vi "MB test.vi"() -> ()   [LabVIEW 2021]
uses:
  enums/DO.ctl
  enums/Param_MB test.lvlib
  enums/AO.ctl
  Inputs/Inputs.lvlib
  <vilib>/Platform/TimedLoop/XDataNode/XDataNode.xnode
  <vilib>/Platform/TimedLoop/XDataNode/nitl_modes.ctl
  <vilib>/Platform/TimedLoop/XDataNode/XDNodeRunTimeDep.lvlib
  <vilib>/Platform/TimedLoop/XDataNode/wakeup.ctl
  <vilib>/Platform/TimedLoop/XDataNode/timing_clust.ctl
  enums/AI.ctl
  enums/PAR.ctl
  enums/DI.ctl
  enums/DI_FAST.ctl
  enums/ALR.ctl
  enums/System.ctl
  enums/main_prog_state.ctl
  enums/KFM.ctl
  Userlib.lvlib
  OPC/OPC addons.lvlib
  Messages/Messages.lvlib
  enums/REG.ctl
  enums/supervisor_state.ctl
  Alarms/Alarms.lvlib
  enums/init_state.ctl
  enums/close_state.ctl
  MB/Modbus Master CR.lvclass
  PostgreSQL/Save messages PGserver/Save messages PGserver.lvclass
  Modbus_v121c/Data Model/Device Data Model.lvclass
panel:
  in  "DO2D":bool[][](array[boolean])
  in  "AOint":u16[][](array[numeric])
  out "Connect":bool[](array[boolean])
  in  "input Flags":T1={"write database started"=FALSE, "main prog started"=TRUE}
  out "output Flags":T2
  out "comm error":errorcluster
  out "initialise error":errorcluster
  in  "object_name":string="GM1"
  in  "EP_dist":bool
  in  "EP_on":bool
  in  "tick":i64=100 caption="Время цикла основной программы" min=5 max=500 step=1
  in  "stop":bool
  in  "On":bool=TRUE
  # "Включение записи !"
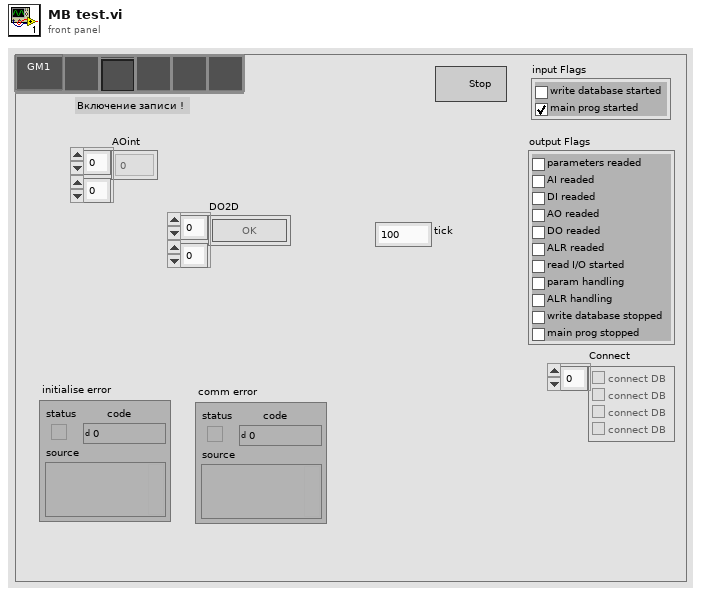
[diagram p1: front panel]
types:
  T1 = cluster{"write database started":bool, "main prog started":bool}
  T2 = cluster{"parameters readed ":bool, "AI readed":bool, "DI readed":bool, "AO readed":bool, "DO readed":bool, "ALR readed":bool, "read I/O started":bool, "param handling":bool, "ALR handling":bool, "write database stopped":bool, "main prog stopped":bool}
  T3 = typedef "Param_MB test.lvlib/init_state.ctl" = enum16{"Init Data", "Init TMPs", "Init system DB", "Init data DB", "Read Enums", "Init arrays", "Init KFM", "Init Param", "Init AI param", "Init DI param", "Init AO param", "Init DO param", "Init ALR param", "Init save progs", "Read OPC param", "Init Shared Variables", "Init regulators", "Init heaters", "Init Y defs", "Exit"}
  T4 = typedef "Param_MB test.lvlib/supervisor_state.ctl" = enum8{"initialize", "read parameters", "read AI param", "read DI param", "read AO param", "read DO param", "read ALR param", "write initialise param", "start read I/O modules", "wait for I/O start", "start param handling", "start ALR handling", "start write database", "start controls", "enable write outputs", "on", "off start", "disable write outputs", "stop controls", "stop write database", "wait for database stopped", "stop ALR handling", "stop param handling", "stop main prog", "stop read I/O modules", "wait for IO stop", "reset", "stop"}
  T5 = typedef "Param_MB test.lvlib/main_prog_state.ctl" = enum16{"Read_AI_Param", "Read_DI_Param", "Read_AO_Param", "Read_DO_Param", "Read_ALR_ON_OFF", "Read_ALR_Param", "Read_Param", "Read_REG_Param", "Timers", "AI", "DI", "SendAItoScada", "SendDItoScada", "Alarms", "SendAItoDB", "SendDItoDB", "SendALRtoDB", "Messages", "Controls", "Control HT1", "QN_control", "QN", "QN_state", "Control EB3", "Outputs", "Exit"}
  T6 = cluster{"KFM":string[], "PAR":string[], "AI":string[], "DI":string[], "DI_fast":string[], "AO":string[], "Regs":string[], "DO":string[], "ALR":string[], "System":string[]}
  T7 = cluster{"object_name":string, "Enums":cluster{"KFM":string[], "PAR":string[], "AI":string[], "DI":string[], "DI_fast":string[], "AO":string[], "Regs":string[], "DO":string[], "ALR":string[], "System":string[]}, "MBs":refnum<class "Modbus Master CR.lvclass">[]}
  T8 = cluster{"current time":timestamp, "Timer_1s":bool, "Timer_10s":bool, "Timer_1day":bool}
  T9 = typedef "Param_MB test.lvlib/REG.ctl" = enum16{"GM1QN1", "GM1QN2", "GM1QN3", "GM1QN4", "GM1QN5", "GM1QN6", "GM1QN7", "GM1QN8", "GM1QN9", "GM1QN10", "GM1QN11", "GM1QN12", "GM1QN13", "GM1QN14", "GM1QN15", "GM1QN16", "GM1QN17", "GM1QN18", "GM1QN19", "GM1QN20", "GM1QN21", "GM1QN22", "GM1QN23"}
  T10 = typedef "Param_MB test.lvlib/System.ctl" = enum16{"GM3HT1", "GM3HT2", "EB2TB1", "EB2TB2", "EB2TB3", "EB3TB1", "EB3TB2", "EB3TB3"}
  T11 = typedef "Param_MB test.lvlib/ALR.ctl" = enum16{"GM1BP1XQ01_H", "GM1BP1XQ01_HH", "GM1BP1XQ01_L", "GM1BP1XQ01_LL", "GM1BP1XQ01_SERR", "GM1BP2XQ01_H", "GM1BP2XQ01_HH", "GM1BP2XQ01_L", "GM1BP2XQ01_LL", "GM1BP2XQ01_SERR", "GM1BP3XQ01_H", "GM1BP3XQ01_HH", "GM1BP3XQ01_L", "GM1BP3XQ01_LL", "GM1BP3XQ01_SERR", "GM1BP4XQ01_H", "GM1BP4XQ01_HH", "GM1BP4XQ01_L", "GM1BP4XQ01_LL", "GM1BP4XQ01_SERR", "GM1BP5XQ01_H", "GM1BP5XQ01_HH", "GM1BP5XQ01_L", "GM1BP5XQ01_LL", "GM1BP5XQ01_SERR", "GM1BP6XQ01_H", "GM1BP6XQ01_HH", "GM1BP6XQ01_L", "GM1BP6XQ01_LL", "GM1BP6XQ01_SERR", "GM1BT1XQ01_H", "GM1BT1XQ01_HH", "GM1BT1XQ01_L", "GM1BT1XQ01_SERR", "GM1BT2XQ01_H", "GM1BT2XQ01_HH", "GM1BT2XQ01_L", "GM1BT2XQ01_SERR", "GM1BT3XQ01_H", "GM1BT3XQ01_HH", "GM1BT3XQ01_L", "GM1BT3XQ01_SERR", "GM1BT4XQ01_H", "GM1BT4XQ01_HH", "GM1BT4XQ01_L", "GM1BT4XQ01_SERR", "GM1BT5XQ01_H", "GM1BT5XQ01_HH", "GM1BT5XQ01_L", "GM1BT5XQ01_SERR", "GM1BT6XQ01_H", "GM1BT6XQ01_HH", "GM1BT6XQ01_L", "GM1BT6XQ01_SERR", "GM1BT7XQ01_H", "GM1BT7XQ01_HH", "GM1BT7XQ01_L", "GM1BT7XQ01_SERR", "GM1BT8XQ01_H", "GM1BT8XQ01_HH", "GM1BT8XQ01_L", "GM1BT8XQ01_SERR", "GM1BT9XQ01_H", "GM1BT9XQ01_HH", "GM1BT9XQ01_L", "GM1BT9XQ01_SERR", "GM1BT10XQ01_H", "GM1BT10XQ01_HH", "GM1BT10XQ01_L", "GM1BT10XQ01_SERR", "GM1BT19XQ01_H", "GM1BT19XQ01_HH", "GM1BT19XQ01_L", "GM1BT19XQ01_SERR", "GM1BT20XQ01_H", "GM1BT20XQ01_HH", "GM1BT20XQ01_L", "GM1BT20XQ01_SERR", "GM1BT21XQ01_H", "GM1BT21XQ01_HH", "GM1BT21XQ01_L", "GM1BT21XQ01_SERR", "GM1BT22XQ01_H", "GM1BT22XQ01_HH", "GM1BT22XQ01_L", "GM1BT22XQ01_SERR", "GM1QN1XQ01_SERR", "GM1QN1XQ02_HH", "GM1QN2XQ01_SERR", "GM1QN2XQ02_HH", "GM1QN3XQ01_SERR", "GM1QN3XQ02_HH", "GM1QN4XQ01_SERR", "GM1QN4XQ02_HH", "GM1QN5XQ01_SERR", "GM1QN5XQ02_HH", "GM1QN6XQ01_SERR", "GM1QN6XQ02_HH", "GM1QN7XQ01_SERR", "GM1QN7XQ02_HH", "GM1QN8XQ01_SERR", "GM1QN8XQ02_HH", "GM1QN9XQ01_SERR", "GM1QN9XQ02_HH", "GM1QN10XQ01_SERR", "GM1QN10XQ02_HH", "GM1QN11XQ01_SERR", "GM1QN11XQ02_HH", "GM1QN12XQ01_SERR", "GM1QN12XQ02_HH", "GM1QN13XQ01_SERR", "GM1QN13XQ02_HH", "GM1QN14XQ01_SERR", "GM1QN14XQ02_HH", "GM1QN15XQ01_SERR", "GM1QN15XQ02_HH", "GM1QN16XQ01_SERR", "GM1QN16XQ02_HH", "GM1QN17XQ01_SERR", "GM1QN17XQ02_HH", "GM1QN18XQ01_SERR", "GM1QN18XQ02_HH", "GM1QN19XQ01_SERR", "GM1QN19XQ02_HH", "GM1QN20XQ01_SERR", "GM1QN20XQ02_HH", "GM1QN21XQ01_SERR", "GM1QN21XQ02_HH", "GM1QN22XQ01_SERR", "GM1QN22XQ02_HH", "GM1QN23XQ01_SERR", "GM1QN23XQ02_HH", "HX1BT11XQ01_H", "HX1BT11XQ01_HH", "HX1BT11XQ01_L", "HX1BT11XQ01_SERR", "HX1BT12XQ01_H", "HX1BT12XQ01_HH", "HX1BT12XQ01_L", "HX1BT12XQ01_SERR", "HX1BT21XQ01_H", "HX1BT21XQ01_HH", "HX1BT21XQ01_L", "HX1BT21XQ01_SERR", "HX1BT22XQ01_H", "HX1BT22XQ01_HH", "HX1BT22XQ01_L", "HX1BT22XQ01_SERR", "HX1BT31XQ01_H", "HX1BT31XQ01_HH", "HX1BT31XQ01_L", "HX1BT31XQ01_SERR", "HX1BT32XQ01_H", "HX1BT32XQ01_HH", "HX1BT32XQ01_L", "HX1BT32XQ01_SERR", "HX1BT41XQ01_H", "HX1BT41XQ01_HH", "HX1BT41XQ01_L", "HX1BT41XQ01_SERR", "HX1BT42XQ01_H", "HX1BT42XQ01_HH", "HX1BT42XQ01_L", "HX1BT42XQ01_SERR", "GM1JBA1JA1_CONN", "GM1JBA1JA2_CONN", "GM1JBA2JA1_CONN", "GM1JBA2JA2_CONN", "GM1JBA3JA1_CONN", "HX1KF1A16_CONN", "HX1KF1A17_CONN", "GM1KF1A18_CONN"}
  T12 = typedef "Param_MB test.lvlib/DO.ctl" = enum16{"GM1FZ1_YB47"}
  T13 = typedef "Param_MB test.lvlib/AO.ctl" = enum16{"GM1QN1_YQ01", "GM1QN2_YQ01", "GM1QN3_YQ01", "GM1QN4_YQ01", "GM1QN5_YQ01", "GM1QN6_YQ01", "GM1QN7_YQ01", "GM1QN8_YQ01", "GM1QN9_YQ01", "GM1QN10_YQ01", "GM1QN11_YQ01", "GM1QN12_YQ01", "GM1QN13_YQ01", "GM1QN14_YQ01", "GM1QN15_YQ01", "GM1QN16_YQ01", "GM1QN17_YQ01", "GM1QN18_YQ01", "GM1QN19_YQ01", "GM1QN20_YQ01", "GM1QN21_YQ01", "GM1QN22_YQ01", "GM1QN23_YQ01"}
  T14 = typedef "Param_MB test.lvlib/DI_FAST.ctl" = enum16{"W1.KF_XB01", "W1.KF_XB02", "W1.KF_XB03", "W1.KF_XB04", "W1.KF_XB05", "W1.KF_XB06", "W1.KF_XB07", "W1.KF_XB08", "W1.KF_XB09", "W1.KF_XB10", "W1.KF_XB11", "W1.KF_XB12", "W1.KF_XB13", "W1.KF_XB14", "W1.KF_XB15", "W1.KF_XB16"}
  T15 = typedef "Param_MB test.lvlib/DI.ctl" = enum16{"GM1FZ1_XB19"}
  T16 = typedef "Param_MB test.lvlib/AI.ctl" = enum16{"GM1BP1_XQ01", "GM1BP2_XQ01", "GM1BP3_XQ01", "GM1BP4_XQ01", "GM1BP5_XQ01", "GM1BP6_XQ01", "GM1BT1_XQ01", "GM1BT2_XQ01", "GM1BT3_XQ01", "GM1BT4_XQ01", "GM1BT5_XQ01", "GM1BT6_XQ01", "GM1BT7_XQ01", "GM1BT8_XQ01", "GM1BT9_XQ01", "GM1BT10_XQ01", "GM1BT19_XQ01", "GM1BT20_XQ01", "HX1BT11_XQ01", "HX1BT12_XQ01", "HX1BT21_XQ01", "HX1BT22_XQ01", "HX1BT31_XQ01", "HX1BT32_XQ01", "HX1BT41_XQ01", "HX1BT42_XQ01", "GM1QN1_XQ01", "GM1QN2_XQ01", "GM1QN3_XQ01", "GM1QN4_XQ01", "GM1QN5_XQ01", "GM1QN6_XQ01", "GM1QN7_XQ01", "GM1QN8_XQ01", "GM1QN9_XQ01", "GM1QN10_XQ01", "GM1QN11_XQ01", "GM1QN12_XQ01", "GM1QN13_XQ01", "GM1QN14_XQ01", "GM1QN15_XQ01", "GM1QN16_XQ01", "GM1QN17_XQ01", "GM1QN18_XQ01", "GM1QN19_XQ01", "GM1QN20_XQ01", "GM1QN21_XQ01", "GM1QN22_XQ01", "GM1QN23_XQ01", "GM1QN1_XQ02", "GM1QN2_XQ02", "GM1QN3_XQ02", "GM1QN4_XQ02", "GM1QN5_XQ02", "GM1QN6_XQ02", "GM1QN7_XQ02", "GM1QN8_XQ02", "GM1QN9_XQ02", "GM1QN10_XQ02", "GM1QN11_XQ02", "GM1QN12_XQ02", "GM1QN13_XQ02", "GM1QN14_XQ02", "GM1QN15_XQ02", "GM1QN16_XQ02", "GM1QN17_XQ02", "GM1QN18_XQ02", "GM1QN19_XQ02", "GM1QN20_XQ02", "GM1QN21_XQ02", "GM1QN22_XQ02", "GM1QN23_XQ02", "GM1BT21_XQ01", "GM1BT22_XQ01"}
  T17 = typedef "Param_MB test.lvlib/PAR.ctl" = enum16{"GM1QN1_alr_value", "GM1QN1_auto_value", "GM1QN1_output_set_time", "GM1QN1_group", "GM1QN1_process_gas", "GM1QN2_alr_value", "GM1QN2_auto_value", "GM1QN2_output_set_time", "GM1QN2_group", "GM1QN2_process_gas", "GM1QN3_alr_value", "GM1QN3_auto_value", "GM1QN3_output_set_time", "GM1QN3_group", "GM1QN3_process_gas", "GM1QN4_alr_value", "GM1QN4_auto_value", "GM1QN4_output_set_time", "GM1QN4_group", "GM1QN4_process_gas", "GM1QN5_alr_value", "GM1QN5_auto_value", "GM1QN5_output_set_time", "GM1QN5_group", "GM1QN5_process_gas", "GM1QN6_alr_value", "GM1QN6_auto_value", "GM1QN6_output_set_time", "GM1QN6_group", "GM1QN6_process_gas", "GM1QN7_alr_value", "GM1QN7_auto_value", "GM1QN7_output_set_time", "GM1QN7_group", "GM1QN7_process_gas", "GM1QN8_alr_value", "GM1QN8_auto_value", "GM1QN8_output_set_time", "GM1QN8_group", "GM1QN8_process_gas", "GM1QN9_alr_value", "GM1QN9_auto_value", "GM1QN9_output_set_time", "GM1QN9_group", "GM1QN9_process_gas", "GM1QN10_alr_value", "GM1QN10_auto_value", "GM1QN10_output_set_time", "GM1QN10_group", "GM1QN10_process_gas", "GM1QN11_alr_value", "GM1QN11_auto_value", "GM1QN11_output_set_time", "GM1QN11_group", "GM1QN11_process_gas", "GM1QN12_alr_value", "GM1QN12_auto_value", "GM1QN12_output_set_time", "GM1QN12_group", "GM1QN12_process_gas", "GM1QN13_alr_value", "GM1QN13_auto_value", "GM1QN13_output_set_time", "GM1QN13_group", "GM1QN13_process_gas", "GM1QN14_alr_value", "GM1QN14_auto_value", "GM1QN14_output_set_time", "GM1QN14_group", "GM1QN14_process_gas", "GM1QN15_alr_value", "GM1QN15_auto_value", "GM1QN15_output_set_time", "GM1QN15_group", "GM1QN15_process_gas", "GM1QN16_alr_value", "GM1QN16_auto_value", "GM1QN16_output_set_time", "GM1QN16_group", "GM1QN16_process_gas", "GM1QN17_alr_value", "GM1QN17_auto_value", "GM1QN17_output_set_time", "GM1QN17_group", "GM1QN17_process_gas", "GM1QN18_alr_value", "GM1QN18_auto_value", "GM1QN18_output_set_time", "GM1QN18_group", "GM1QN18_process_gas", "GM1QN19_alr_value", "GM1QN19_auto_value", "GM1QN19_output_set_time", "GM1QN19_group", "GM1QN19_process_gas", "GM1QN20_alr_value", "GM1QN20_auto_value", "GM1QN20_output_set_time", "GM1QN20_group", "GM1QN20_process_gas", "GM1QN21_alr_value", "GM1QN21_auto_value", "GM1QN21_output_set_time", "GM1QN21_group", "GM1QN21_process_gas", "GM1QN22_alr_value", "GM1QN22_auto_value", "GM1QN22_output_set_time", "GM1QN22_group", "GM1QN22_process_gas", "GM1QN23_alr_value", "GM1QN23_auto_value", "GM1QN23_output_set_time", "GM1QN23_group", "GM1QN23_process_gas"}
  T18 = typedef "Param_MB test.lvlib/KFM.ctl" = enum16{"GM1KF1_A1", "GM1JBA1_JA1", "GM1JBA1_JA2", "GM1JBA2_JA1", "GM1JBA2_JA2", "GM1JBA3_JA1", "HX1KF1_A16", "HX1KF1_A17", "GM1KF1_A18"}
  T19 = typedef "XDNodeRunTimeDep.lvlib/timing_clust.ctl" = cluster{"Expected End [f-1]":u64, "Actual End [f-1]":u64, "Finished Late? [f-1]":bool, "Expected End [i-1]":u64, "Actual End [i-1]":u64, "Finished Late? [i-1]":bool, "Expected Start [i]":u64, "Actual Start [i]":u64, "Expected Start [f]":u64, "Actual Start [f]":u64, "Source Name":string, "Structure Name":string, "Period":i64, "Deadline":i64, "Offset":i64, "Start":i64, "Priority":i32, "Timeout":i32, "Mode":T20, "Wakeup Reason":T21, "Error":errorcluster, "Source Type":string, "Secondary Source Type":string, "Global End Time":u64, "Global Start Time":u64, "Frame Duration":u64, "Iteration Duration":u64, "Assigned CPU":i32, "I/O Scan Engine Mode":u32}
  T20 = typedef "XDNodeRunTimeDep.lvlib/nitl_modes.ctl" = enum32{"No Change", "Process missed periods, maintain original phase", "Discard missed periods, maintain original phase", "Process missed periods, ignore original phase", "Discard missed periods, ignore original phase"}
  T21 = typedef "XDNodeRunTimeDep.lvlib/wakeup.ctl" = enum32{"Normal", "Aborted", "Asynchronous wakeup", "Timing source error", "Timed loop error", "Timeout"}
  T22 = typedef "MB_v2.lvlib/Modbus Master CR.lvclass/N channel.ctl" = cluster{"N DI channel":u16, "N DO channel":u16, "N AI channel":u16, "N AO channel":u16}
  T23 = typedef "Param_MB test.lvlib/close_state.ctl" = enum16{"QN_state notifier", "QN_control_queue", "ALR notifires", "ALR", "DO notifires", "DO", "AO notifires", "AO", "DI notifres", "DI", "AI notifires", "AI", "OPC", "Param", "SaveMessageProg", "KFM DadaRef", "KFM Registers", "KFM StatusRef", "Exit"}
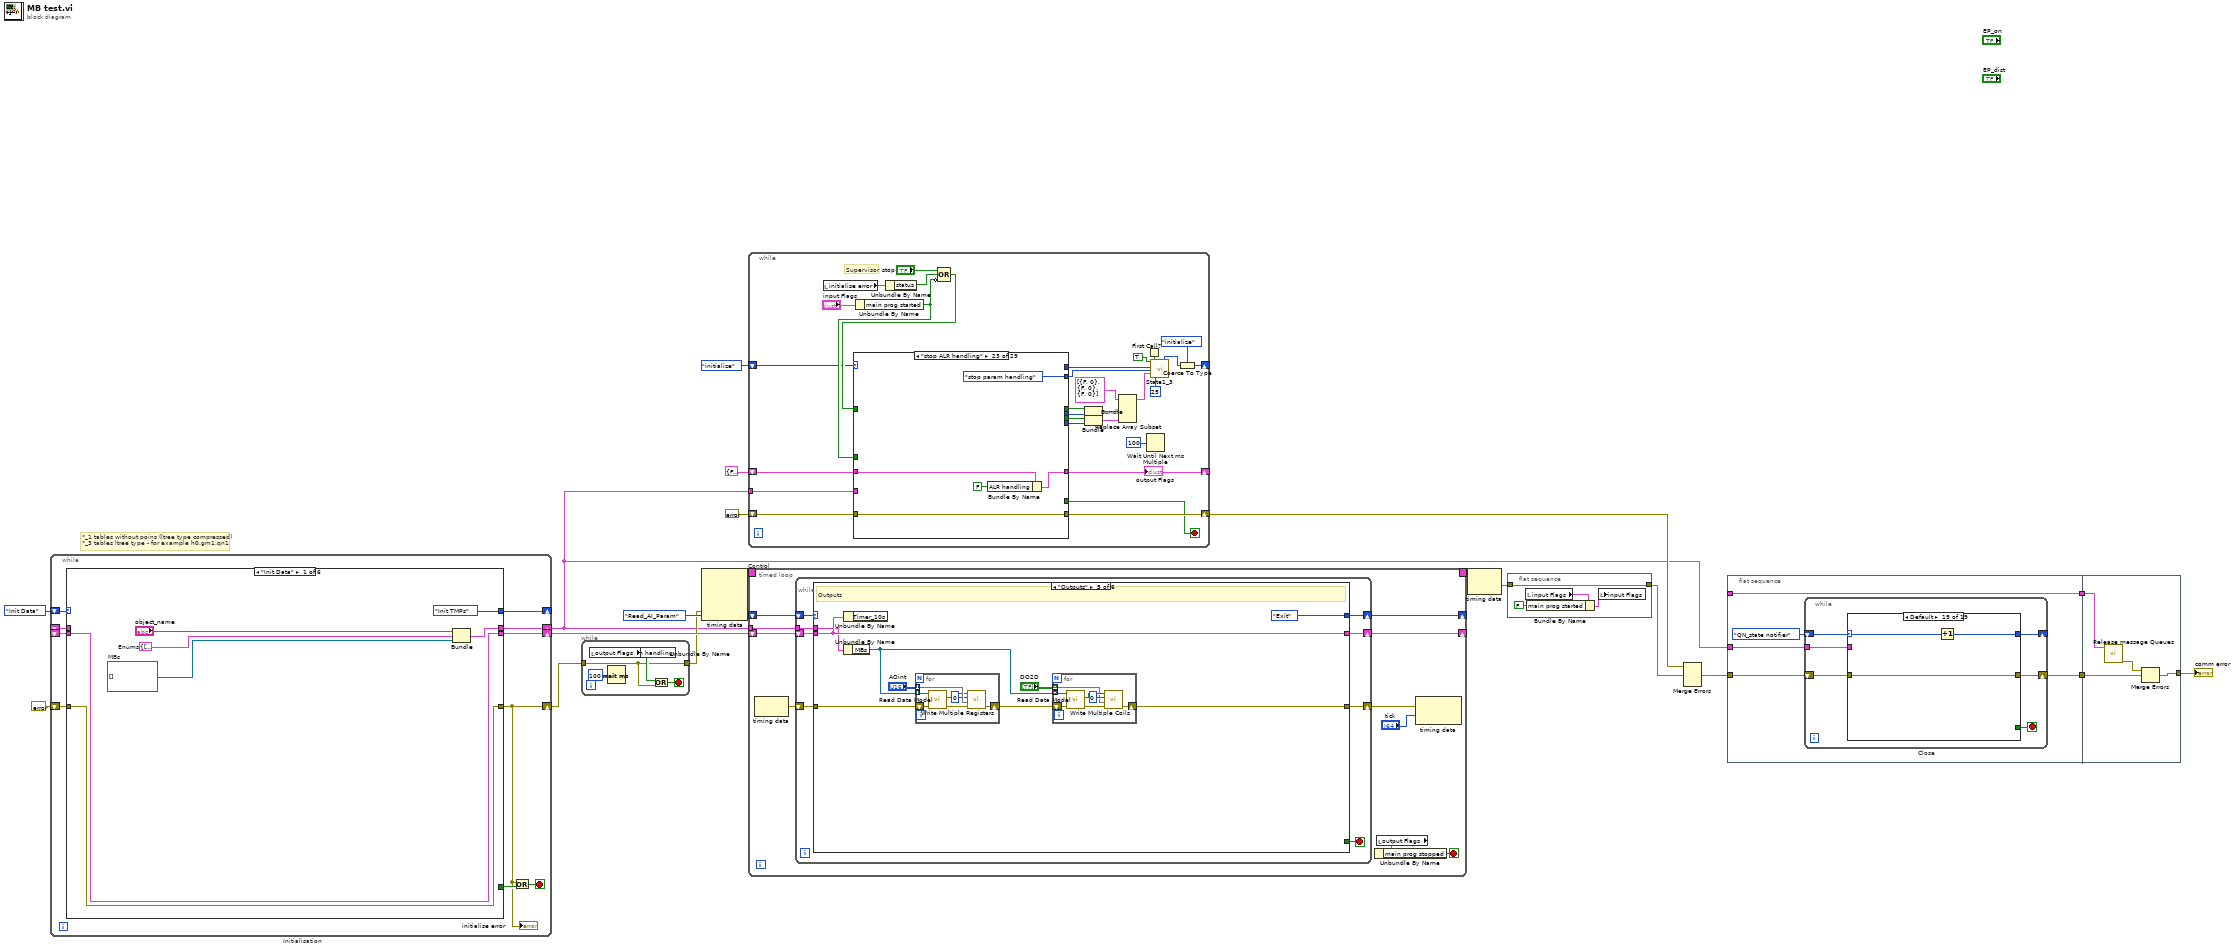
[diagram p0: block diagram]
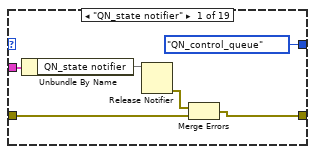
[diagram p2: hidden frame]
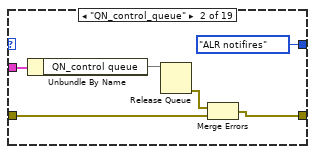
[diagram p3: hidden frame]
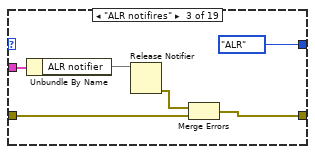
[diagram p4: hidden frame]
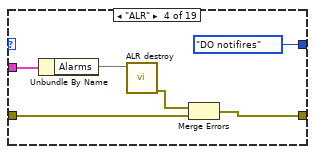
[diagram p5: hidden frame]
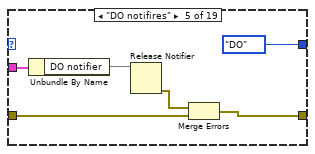
[diagram p6: hidden frame]
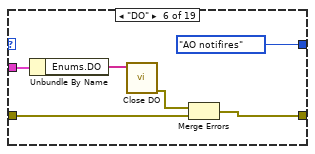
[diagram p7: hidden frame]
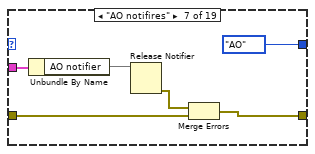
[diagram p8: hidden frame]
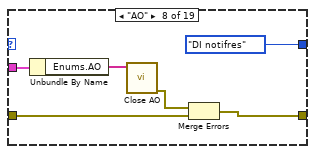
[diagram p9: hidden frame]
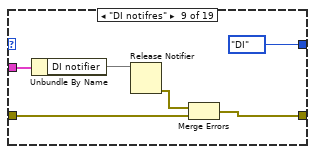
[diagram p10: hidden frame]
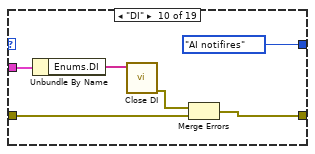
[diagram p11: hidden frame]
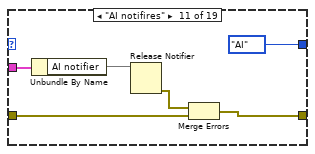
[diagram p12: hidden frame]
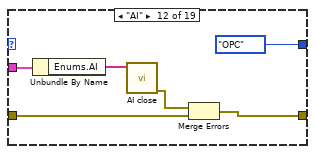
[diagram p13: hidden frame]
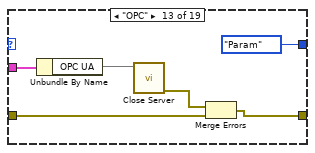
[diagram p14: hidden frame]
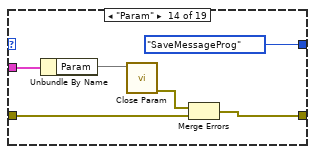
[diagram p15: hidden frame]
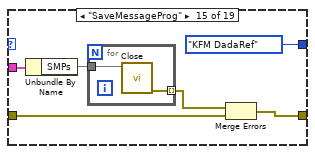
[diagram p16: hidden frame]
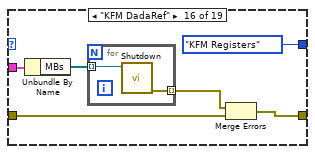
[diagram p17: hidden frame]
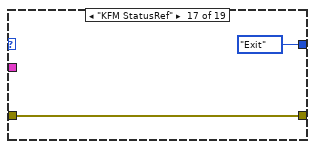
[diagram p18: hidden frame]
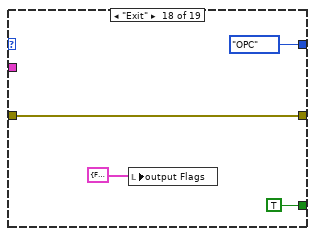
[diagram p19: hidden frame]
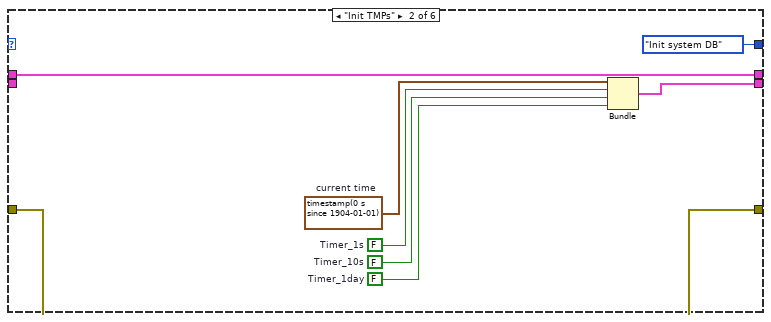
[diagram p20: hidden frame]
diagram:
  # "*_1 tables without poins (ltree type compressed)\n*_3 tables ltree type - for example h0.gm1.qn1"
  n1 = while "Initialisation" {
    shift-right: [w20] -> w9
    shift-left: errorcluster {"status"=FALSE, "code"=0, "source"=""} ("error out") -> [w26]
    shift-right: [w29] -> w2
    shift-left: _ -> [w27]
    shift-right: [w25] -> _
    shift-left: init_state."Init Data" -> [w28]
    shift-right: [w22] -> w10
    shift-left: _ -> [w21]
    stop <- w23 stop-if-true
    # "Initialisation"
    n2 = case shown="\"Init Data\"" w28 {
      tunnel: [w34 w43 w61 w83 w101 w104] -> w20
      selector: w28 -> [_ _ _ _ _ w107]
      tunnel: [w35 w42 w78 w88 w102 w105] -> w29
      tunnel: w27 -> [_ w42 w79 w87 w102 w105]
      tunnel: w26 -> [w34 w43 w45 w84 w101 w104]
      tunnel: [init_state."Init TMPs" init_state."Init system DB" init_state."Init arrays" init_state."Init Param" init_state."Init Data" w106] -> w25
      tunnel: [_ _ _ _ TRUE _] -> w24
      tunnel: [w32 w41 w81 w94 w99 w108] -> w22
      tunnel: w21 -> [w32 _ w81 w94 w99 w108]
      frame "Init Data" {
        w30 = refnum<class "Modbus Master CR.lvclass">[] []  # MBs
        w33 = T6 {"KFM"=[], "PAR"=[], "AI"=[], "DI"=[], "DI_fast"=[], "AO"=[], "Regs"=[], "DO"=[], "ALR"=[], "System"=[]}  # Enums
        n3 = Bundle("object_name"="object_name", "Enums"=w33, "MBs"=w30) -> (w35:T7)  [unwired: 1 in]
      }
      frame "Init TMPs" {
        w37 = FALSE  # Timer_10s
        w38 = FALSE  # Timer_1day
        w39 = FALSE  # Timer_1s
        w40 = timestamp(0 s since 1904-01-01)  # current time
        n4 = Bundle("current time"=w40, "Timer_1s"=w39, "Timer_10s"=w37, "Timer_1day"=w38) -> (w41:T8)  [unwired: 1 in]
      }
      frame "Read Enums" {
        w47 = REG."GM1QN1"  # REG
        w50 = T6 {"KFM"=[], "PAR"=[], "AI"=[], "DI"=[], "DI_fast"=[], "AO"=[], "Regs"=[], "DO"=[], "ALR"=[], "System"=[]}  # Enums
        w52 = System."GM3HT1"  # System_enum
        w53 = ALR."GM1JBA1JA1_CONN"  # ALR_enum
        w54 = DO."GM1FZ1_YB47"  # DO_enum
        w55 = AO."GM1QN1_YQ01"  # AO_enum
        w56 = DI_FAST."W1.KF_XB01"  # DI_enum fast
        w57 = DI."GM1FZ1_XB19"  # DI_enum
        w58 = AI."GM1QN1_XQ01"  # AI_enum
        w59 = PAR."GM1QN1_output_set_time"  # PAR_enum
        w60 = KFM."GM1JBA1_JA1"  # KFM_enum
        # "компьютер на 0 месте"
        n5 = call <userlib>:"Get Strings from Enum__ogtk.vi"("error in (no error)"=w45, "Enum"=w60) -> ("error out"=w70:errorcluster, "Enum Strings"=w77:string[])  [unwired: 6 in, 2 out]
        n6 = call <userlib>:"Get Strings from Enum__ogtk.vi"("error in (no error)"=w45, "Enum"=w59) -> ("error out"=w69:errorcluster, "Enum Strings"=w76:string[])  [unwired: 6 in, 2 out]
        n7 = call <userlib>:"Get Strings from Enum__ogtk.vi"("error in (no error)"=w45, "Enum"=w58) -> ("error out"=w68:errorcluster, "Enum Strings"=w75:string[])  [unwired: 6 in, 2 out]
        n8 = call <userlib>:"Get Strings from Enum__ogtk.vi"("error in (no error)"=w45, "Enum"=w57) -> ("error out"=w67:errorcluster, "Enum Strings"=w74:string[])  [unwired: 6 in, 2 out]
        n9 = call <userlib>:"Get Strings from Enum__ogtk.vi"("error in (no error)"=w45, "Enum"=w56) -> ("error out"=w66:errorcluster, "Enum Strings"=w73:string[])  [unwired: 6 in, 2 out]
        n10 = call <userlib>:"Get Strings from Enum__ogtk.vi"("error in (no error)"=w45, "Enum"=w55) -> ("error out"=w65:errorcluster, "Enum Strings"=w72:string[])  [unwired: 6 in, 2 out]
        n11 = call <userlib>:"Get Strings from Enum__ogtk.vi"("error in (no error)"=w45, "Enum"=w47) -> ("Enum Strings"=w46:string[])  [unwired: 6 in, 3 out]
        n12 = call <userlib>:"Get Strings from Enum__ogtk.vi"("error in (no error)"=w45, "Enum"=w54) -> ("error out"=w64:errorcluster, "Enum Strings"=w48:string[])  [unwired: 6 in, 2 out]
        n13 = call <userlib>:"Get Strings from Enum__ogtk.vi"("error in (no error)"=w45, "Enum"=w53) -> ("error out"=w63:errorcluster, "Enum Strings"=w71:string[])  [unwired: 6 in, 2 out]
        n14 = call <userlib>:"Get Strings from Enum__ogtk.vi"("error in (no error)"=w45, "Enum"=w52) -> ("error out"=w62:errorcluster)  [unwired: 6 in, 3 out]
        n15 = Bundle By Name(cluster=w50, "KFM"=w77, "PAR"=w76, "AI"=w75, "DI"=w74, "DI_fast"=w73, "AO"=w72, "Regs"=w46, "DO"=w48, "ALR"=w71, "System"=string[] []) -> (w49:T6)
        n16 = Merge Errors(w70, w69, w68, w67, w66, w65, w64, w63, w62) -> (w61:errorcluster)
        n17 = Bundle By Name(cluster=w79, "Enums"=w49) -> (w78:T7)
      }
      frame "Init KFM" {
        n18 = Unbundle By Name(w87) -> ("Enums.KFM"=w91:string[])
        n19 = call "init classes.vi"("error in (no error)"=w84, "MVINames"=string[] []) -> ("error out"=w93:errorcluster, "MBs"=w85:refnum<class "Modbus Master CR.lvclass">[])  [unwired: 8 in]
        n20 = call "MB Param redefine.vi"("error in (no error)"=w93, "KFMTable"="kfm_1", "KFM param"=w91, "MBs"=w85) -> ("error"=w92:errorcluster, "MBs out"=w89:refnum<class "Modbus Master CR.lvclass">[])  [unwired: 6 in]
        n21 = call "Start read modules.vi"("error in"=w92, "classes"=w89) -> ("error out"=w83:errorcluster, "classes initialised"=w86:refnum<class "Modbus Master CR.lvclass">[])  [unwired: 8 in]
        n22 = Bundle By Name(cluster=w87, "MBs"=w86) -> (w88:T7)
      }
      frame "Exit" {
        n23 = local read "input Flags"() -> (w98:T1)
        n24 = Bundle By Name(cluster=w98, "main prog started"=TRUE) -> (w97:T1)
        n25 = local write "input Flags"(w97) -> ()
      }
      frame Default {
        n26 = Increment(x=w107) -> (x+1=w106:T3)
      }
    }
    "initialise error" <- w20
    n27 = Or(x=w20, y=w24) -> (x .or. y?=w23:bool)
  }
  n28 = while {
    tunnel: w9 -> [w110]
    tunnel: [w110] -> w8
    stop <- w109 stop-if-true
    n29 = local read "output Flags"() -> (w113:T2)
    n30 = Wait (ms)(milliseconds to wait=u32 100) -> ()  [unwired: 1 out]
    n31 = Unbundle By Name(w113) -> ("param handling"=w112:bool)
    n32 = Or(x=w112, y=w110) -> (x .or. y?=w109:bool)
  }
  n33 = node-c288(w8) -> (w19:T19)  [unwired: 3 in]
  n34 = while {
    tunnel: w2 -> [w125]
    shift-right: [w121] -> _
    shift-left: T2 {"parameters readed "=FALSE, "AI readed"=FALSE, "DI readed"=FALSE, "AO readed"=FALSE, "DO readed"=FALSE, "ALR readed"=FALSE, "read I/O started"=FALSE, "param handling"=FALSE, "ALR handling"=FALSE, "write database stopped"=FALSE, "main prog stopped"=FALSE} ("output Flags") -> [w126]
    shift-right: [w123] -> w7
    shift-left: errorcluster {"status"=FALSE, "code"=0, "source"=""} ("error out") -> [w124]
    shift-right: [w132] -> _
    shift-left: supervisor_state."initialize" ("Z2(SetState)") -> [w114]
    stop <- w122 stop-if-true
    # "Supervisor"
    n35 = local read "initialise error"() -> (w130:errorcluster)
    n36 = Unbundle By Name("input Flags") -> ("main prog started"=w127:bool)
    n37 = Unbundle By Name(w130) -> ("status"=w142:bool)
    n38 = Compound Arithmetic op=OR("stop", w142, invert w127) -> (w128:bool)
    n39 = case shown="\"stop ALR handling\"" w114 {
      selector: w114 -> [w145 _ _ _ _ _ _ _ _ _ _ _ _ _ _ _ _ _ _ _ _ _ _ _ _ _ _ _ _]
      tunnel: [_ _ w170 w184 w198 w212 w226 w240 _ w256 w275 w283 w290 w299 w305 w314 w328 _ _ _ _ _ _ _ _ _ _ _ _] -> w117
      tunnel: [_ _ supervisor_state."off start" ("Z2(SetState)") supervisor_state."off start" ("Z2(SetState)") supervisor_state."off start" ("Z2(SetState)") supervisor_state."off start" ("Z2(SetState)") supervisor_state."off start" ("Z2(SetState)") supervisor_state."off start" ("Z2(SetState)") _ supervisor_state."off start" ("Z2(SetState)") supervisor_state."off start" ("Z2(SetState)") supervisor_state."off start" ("Z2(SetState)") supervisor_state."off start" ("Z2(SetState)") supervisor_state."off start" ("Z2(SetState)") supervisor_state."off start" ("Z2(SetState)") supervisor_state."off start" ("Z2(SetState)") supervisor_state."off start" ("Z2(SetState)") _ _ _ _ _ _ _ _ _ _ _ _] -> w118
      tunnel: [u32 0 ("T") u32 0 ("T") u32 60000 ("T") u32 60000 ("T") u32 60000 ("T") u32 60000 ("T") u32 60000 ("T") u32 60000 ("T") _ _ u32 10000 ("T") u32 5000 ("T") _ _ u32 100 ("T") _ _ _ _ _ _ u32 60000 ("T") _ _ _ _ u32 10000 ("T") u32 2000 ("T") _] -> w115
      tunnel: [w144 supervisor_state."read parameters" ("Z2(SetState)") supervisor_state."read AI param" ("Z2(SetState)") supervisor_state."read DI param" ("Z2(SetState)") supervisor_state."read AO param" ("Z2(SetState)") supervisor_state."read DO param" ("Z2(SetState)") supervisor_state."read ALR param" ("Z2(SetState)") supervisor_state."start read I/O modules" ("Z2(SetState)") supervisor_state."start read I/O modules" ("Z2(SetState)") supervisor_state."wait for I/O start" ("Z2(SetState)") supervisor_state."start param handling" ("Z2(SetState)") supervisor_state."start ALR handling" ("Z2(SetState)") supervisor_state."start write database" ("Z2(SetState)") supervisor_state."start controls" ("Z2(SetState)") supervisor_state."enable write outputs" ("Z2(SetState)") supervisor_state."on" ("Z2(SetState)") supervisor_state."on" ("Z2(SetState)") supervisor_state."disable write outputs" ("Z2(SetState)") supervisor_state."stop controls" ("Z2(SetState)") supervisor_state."stop write database" ("Z2(SetState)") w355 w365 supervisor_state."stop param handling" ("Z2(SetState)") supervisor_state."stop main prog" ("Z2(SetState)") supervisor_state."stop main prog" ("Z2(SetState)") supervisor_state."wait for IO stop" ("Z2(SetState)") w398 supervisor_state."stop" ("Z2(SetState)") supervisor_state."stop" ("Z2(SetState)")] -> w116
      tunnel: [_ _ w160 w178 w192 w206 w220 w230 _ _ w267 _ _ _ _ _ _ _ _ _ _ w360 _ _ w381 _ w399 _ _] -> w119
      tunnel: [_ _ supervisor_state."read AI param" ("Z2(SetState)") supervisor_state."read DI param" ("Z2(SetState)") supervisor_state."read AO param" ("Z2(SetState)") supervisor_state."read DO param" ("Z2(SetState)") supervisor_state."read ALR param" ("Z2(SetState)") supervisor_state."start read I/O modules" ("Z2(SetState)") _ _ supervisor_state."start param handling" ("Z2(SetState)") _ _ _ _ _ _ _ _ _ w355 w365 _ _ supervisor_state."stop read I/O modules" ("Z2(SetState)") _ w398 _ _] -> w120
      tunnel: w128 -> [_ _ w170 w184 w198 w212 w226 w240 _ w256 w275 w283 w290 w299 w305 w314 w328 _ _ _ _ _ _ _ _ _ _ _ _]
      tunnel: [w148 w157 w161 w179 w193 w207 w221 w231 w246 w254 w264 w279 w287 w298 w303 w313 w327 w337 w344 w347 w353 w361 w368 w373 w378 w391 w401 w404 w408] -> w121
      tunnel: w126 -> [w148 w157 w163 w181 w195 w209 w223 w235 w246 w254 w263 w278 w286 w298 w303 w313 w327 w337 w344 w347 w353 w362 w367 w372 w377 w391 w401 w404 w408]
      tunnel: w124 -> [w147 w154 w165 w177 w191 w205 w219 w234 w245 w249 w262 w281 w289 w295 w302 w310 w324 w336 w340 w346 w352 w356 w370 w375 w383 w386 w394 w403 w407]
      tunnel: [w147 w150 w164 w175 w190 w204 w217 w232 w245 w247 w259 w281 w289 w294 w302 w308 w320 w336 w341 w346 w350 w359 w370 w375 w383 w385 w393 w403 w407] -> w123
      tunnel: w125 -> [_ w156 w162 w180 w194 w208 w222 w233 _ w255 w272 _ _ w297 _ w312 w325 _ w343 _ w354 w364 _ _ _ w389 w396 _ _]
      tunnel: w127 -> [_ _ _ _ _ _ _ _ _ _ _ _ _ _ _ _ _ _ _ _ _ _ _ _ w380 _ _ _ _]
      tunnel: [_ _ _ _ _ _ _ _ _ _ _ _ _ _ _ _ _ _ _ _ _ _ _ _ _ _ _ _ TRUE] -> w122
      frame Default {
        n40 = Increment(x=w145) -> (x+1=w144:T4)
      }
      frame "initialize" {
        n41 = Unbundle By Name(w156) -> ("MBs"=w155:refnum<class "Modbus Master CR.lvclass">[])
        n42 = call "Send Run.vi"("error in"=w154, "Run"=FALSE, "MBs"=w155) -> ("error out"=w151:errorcluster, "MBs out"=w152:refnum<class "Modbus Master CR.lvclass">[])  [unwired: 7 in]
        n43 = call "Send Write.vi"("error in"=w151, "Write"=FALSE, "MBs"=w152) -> ("error out"=w150:errorcluster)  [unwired: 7 in, 1 out]
      }
      frame "read parameters" {
        n44 = Unbundle By Name(w162) -> ("Param"=w167)
        n45 = call "Read PARinitialised.vi"("error in (no error)"=w165, "PAR in"=w167) -> ("error out"=w164:errorcluster, "initialised"=w166:u8)  [unwired: 7 in, 1 out]
        n46 = case shown="1, Default" w166 {
          tunnel: [_ TRUE] -> w160
          frame 0 {
          }
          frame 1, Default {
          }
        }
        n47 = Bundle By Name(cluster=w163, "parameters readed"=w160) -> (w161:T2)
      }
      frame "read AI param" {
        n48 = Unbundle By Name(w180) -> ("Enums.AI"=w176:string[])
        n49 = call "Read AIinitialised.vi"("error in (no error)"=w177, "AI in"=w176) -> ("error out"=w175:errorcluster, "initialised"=w174:u8)  [unwired: 7 in, 1 out]
        n50 = case shown="1, Default" w174 {
          tunnel: [_ TRUE] -> w178
          frame 0 {
          }
          frame 1, Default {
          }
        }
        n51 = Bundle By Name(cluster=w181, "AI readed"=w178) -> (w179:T2)
      }
      frame "read DI param" {
        n52 = Unbundle By Name(w194) -> ("Enums.DI"=w189:string[])
        n53 = call "Read DIinitialised.vi"("error in (no error)"=w191, "DI in"=w189) -> ("error out"=w190:errorcluster, "initialised"=w188:u8)  [unwired: 7 in, 1 out]
        n54 = case shown="1, Default" w188 {
          tunnel: [_ TRUE] -> w192
          frame 0 {
          }
          frame 1, Default {
          }
        }
        n55 = Bundle By Name(cluster=w195, "DI readed"=w192) -> (w193:T2)
      }
      frame "read AO param" {
        n56 = Unbundle By Name(w208) -> ("Enums.AO"=w202:string[])
        n57 = call "Read AOinitialised.vi"("error in (no error)"=w205, "AO in"=w202) -> ("error out"=w204:errorcluster, "initialised"=w203:u8)  [unwired: 7 in, 1 out]
        n58 = case shown="1, Default" w203 {
          tunnel: [_ TRUE] -> w206
          frame 0 {
          }
          frame 1, Default {
          }
        }
        n59 = Bundle By Name(cluster=w209, "AO readed"=w206) -> (w207:T2)
      }
      frame "read DO param" {
        n60 = Unbundle By Name(w222) -> ("Enums.DO"=w218:string[])
        n61 = call "Read DOinitialised.vi"("error in (no error)"=w219, "DO in"=w218) -> ("error out"=w217:errorcluster, "initialised"=w216:u8)  [unwired: 7 in, 1 out]
        n62 = case shown="1, Default" w216 {
          tunnel: [_ TRUE] -> w220
          frame 0 {
          }
          frame 1, Default {
          }
        }
        n63 = Bundle By Name(cluster=w223, "DO readed"=w220) -> (w221:T2)
      }
      frame "read ALR param" {
        n64 = Unbundle By Name(w233) -> ("Alarms"=w237)
        n65 = call "Read ALRPinitialised.vi"("error in (no error)"=w234, "ALR in"=w237) -> ("error out"=w232:errorcluster, "initialised"=w236:u8)  [unwired: 7 in, 1 out]
        n66 = case shown="1, Default" w236 {
          tunnel: [_ TRUE] -> w230
          frame 0 {
          }
          frame 1, Default {
          }
        }
        n67 = Bundle By Name(cluster=w235, "ALR readed"=w230) -> (w231:T2)
      }
      frame "write initialise param" {
        # "Добавить при необходимости"
      }
      frame "start read I/O modules" {
        n68 = Unbundle By Name(w255) -> ("MBs"=w248:refnum<class "Modbus Master CR.lvclass">[])
        n69 = call "Send Run.vi"("error in"=w249, "Run"=TRUE, "MBs"=w248) -> ("error out"=w251:errorcluster, "MBs out"=w252:refnum<class "Modbus Master CR.lvclass">[])  [unwired: 7 in]
        n70 = call "Send Write.vi"("error in"=w251, "Write"=FALSE, "MBs"=w252) -> ("error out"=w247:errorcluster)  [unwired: 7 in, 1 out]
      }
      frame "wait for I/O start" {
        # "/2"
        n71 = Unbundle By Name(w272) -> ("MBs"=w261:refnum<class "Modbus Master CR.lvclass">[])
        n72 = call "Read connects.vi"("error in (no error)"=w262, "MBs"=w261) -> ("error out"=w259:errorcluster, "connects"=w260:bool[])  [unwired: 7 in, 1 out]
        n73 = Array Size(array=w260) -> (size(s)=w266:i32)
        n74 = Bundle By Name(cluster=w263, "read I/O started"=TRUE) -> (w264:T2)
        n75 = Boolean To (0,1)(Boolean=w260) -> (0, 1=w271:i16[])
        n76 = Logical Shift(y=i16 -1, x=w266) -> (x << y=w268:i32)
        n77 = Add Array Elements(numeric array=w271) -> (sum=w269:i16)
        n78 = Greater?(x=w269, y=w268) -> (0:w267:bool)
      }
      frame "start param handling" {
        n79 = Bundle By Name(cluster=w278, "param handling"=TRUE) -> (w279:T2)
      }
      frame "start ALR handling" {
        n80 = Bundle By Name(cluster=w286, "ALR handling"=TRUE) -> (w287:T2)
      }
      frame "start write database" {
        n81 = Unbundle By Name(w297) -> ("SMPs"=w296)
        n82 = call "Send Run.vi"("error in"=w295, "Run"=TRUE, "MBs"=w296) -> ("error out"=w294:errorcluster)  [unwired: 7 in, 1 out]
      }
      frame "start controls" {
      }
      frame "enable write outputs" {
        n83 = Unbundle By Name(w312) -> ("MBs"=w309:refnum<class "Modbus Master CR.lvclass">[])
        n84 = call "Send Write.vi"("error in"=w310, "Write"="On", "MBs"=w309) -> ("error out"=w308:errorcluster)  [unwired: 7 in, 1 out]
      }
      frame "on" {
        n85 = local read "On"() -> (w319:bool)
        n86 = feedback-in #1(w319) -> ()
        n87 = feedback #1() -> (w326:bool)  [unwired: 1 in]
        n88 = Unbundle By Name(w325) -> ("MBs"=w323:refnum<class "Modbus Master CR.lvclass">[])
        n89 = Exclusive Or(1:w319, 2:w326) -> (0:w322:bool)
        n90 = case shown="True" w322 {
          tunnel: w324 -> [w331 w333]
          tunnel: [w331 w335] -> w318
          tunnel: w323 -> [_ w334]
          tunnel: w319 -> [_ w332]
          frame False {
          }
          frame True {
            n91 = call "Send Write.vi"("error in"=w333, "Write"=w332, "MBs"=w334) -> ("error out"=w335:errorcluster)  [unwired: 7 in, 1 out]
          }
        }
        n92 = Unbundle By Name(w325) -> ("SMPs"=w321)
        n93 = call "Read connects.vi"("error in (no error)"=w318, "SMPs"=w321) -> ("error out"=w320:errorcluster, "connects"=→"Connect":bool[])  [unwired: 7 in, 1 out]
      }
      frame "off start" {
      }
      frame "disable write outputs" {
        n94 = Unbundle By Name(w343) -> ("MBs"=w339:refnum<class "Modbus Master CR.lvclass">[])
        n95 = call "Send Write.vi"("error in"=w340, "Write"=FALSE, "MBs"=w339) -> ("error out"=w341:errorcluster)  [unwired: 7 in, 1 out]
      }
      frame "stop controls" {
      }
      frame "stop write database" {
        w355 = supervisor_state."wait for database stopped" ("Z2(SetState)")
        n96 = Unbundle By Name(w354) -> ("SMPs"=w351)
        n97 = call "Send Stop.vi"("error in"=w352, "Stop"=TRUE, "SMPs"=w351) -> ("error out"=w350:errorcluster)  [unwired: 7 in, 1 out]
      }
      frame "wait for database stopped" {
        w365 = supervisor_state."stop ALR handling" ("Z2(SetState)")
        n98 = Unbundle By Name(w364) -> ("SMPs"=w357)
        n99 = call "Read connects.vi"("error in (no error)"=w356, "SMPs"=w357) -> ("error out"=w359:errorcluster, "connects"=w358:bool[])  [unwired: 7 in, 1 out]
        n100 = Or Array Elements(Boolean array=w358) -> (logical OR=w363:bool)
        n101 = Not(x=w363) -> (.not. x?=w360:bool)
        n102 = Bundle By Name(cluster=w362, "write database stopped"=w360) -> (w361:T2)
      }
      frame "stop ALR handling" {
        n103 = Bundle By Name(cluster=w367, "ALR handling"=FALSE) -> (w368:T2)
      }
      frame "stop param handling" {
        n104 = Bundle By Name(cluster=w372, "param handling"=FALSE) -> (w373:T2)
      }
      frame "stop main prog" {
        n105 = Not(x=w380) -> (.not. x?=w381:bool)
        n106 = Bundle By Name(cluster=w377, "main prog stopped"=TRUE ("main prog started")) -> (w378:T2)
      }
      frame "stop read I/O modules" {
        n107 = Unbundle By Name(w389) -> ("MBs"=w388:refnum<class "Modbus Master CR.lvclass">[])
        n108 = call "Send Stop.vi"("error in"=w386, "Stop"=TRUE ("Run"), "MBs"=w388) -> ("error out"=w385:errorcluster)  [unwired: 7 in, 1 out]
      }
      frame "wait for IO stop" {
        w398 = supervisor_state."reset" ("Z2(SetState)")
        n109 = Unbundle By Name(w396) -> ("MBs"=w395:refnum<class "Modbus Master CR.lvclass">[])
        n110 = call "Read connects.vi"("error in (no error)"=w394, "MBs"=w395) -> ("error out"=w393:errorcluster, "connects"=w392:bool[])  [unwired: 7 in, 1 out]
        n111 = Or Array Elements(Boolean array=w392) -> (logical OR=w400:bool)
        n112 = Not(x=w400) -> (.not. x?=w399:bool)
      }
      frame "reset" {
      }
      frame "stop" {
      }
    }
    "output Flags" <- w121
    n113 = Bundle(w117, "Z2(SetState)"=w118) -> (w138:cluster{bool, "Z2(SetState)":T4})  [unwired: 1 in]
    n114 = Bundle(w119, "Z2(SetState)"=w120) -> (w136:cluster{bool, "Z2(SetState)":T4})  [unwired: 1 in]
    n115 = Replace Array Subset(array=cluster{"C":bool, "NC":u32}[] [{"C"=FALSE, "NC"=0}, {"C"=FALSE, "NC"=0}, {"C"=FALSE, "NC"=0}] ("appended array"), new element #1=w138, new element #2=w136) -> (w137:cluster{"C":bool, "NC":u32}[])  [unwired: 2 in]
    n116 = First Call?() -> (First Call?: T/F=w135:bool)
    n117 = Wait Until Next ms Multiple(millisecond multiple=u32 100) -> ()  [unwired: 1 out]
    n118 = call "State1_3.vi"("Start"=TRUE, "t"=w115, "Nt"=w116, "C_table"=w137, "Reset"=w135, "End step"=u32 25) -> ("N next"=w134:u32)  [unwired: 8 in, 5 out]
    n119 = Coerce To Type(0:w134, 1:supervisor_state."initialize" ("Z2(SetState)")) -> (2:w132:T4)
  }
  n120 = timed-loop "Control" {
    tunnel: w2 -> [w419]
    shift-right: [w417] -> _
    shift-left: w10 -> [w418]
    timing: w19 -> [_]
    timing-out: [_] -> w18
    shift-right: [w414] -> _
    shift-left: main_prog_state."Read_AI_Param" -> [w413]
    stop <- w410 stop-if-true
    n121 = node-c288() -> (w415:errorcluster)  [unwired: 1 in]
    n122 = while {
      tunnel: w419 -> [w427]
      shift-right: [w425] -> w417
      shift-left: w418 -> [w426]
      shift-right: [w420] -> w416
      shift-left: w415 -> [w424]
      shift-right: [w423] -> w414
      shift-left: w413 -> [w422]
      stop <- w421 stop-if-true
      n123 = case shown="\"Outputs\"" w422 {
        tunnel: w424 -> [w428 w451 w475 w491 w512 w531]
        tunnel: w427 -> [_ _ w476 w494 w514 _]
        tunnel: w426 -> [w430 w462 w474 w493 w515 w532]
        tunnel: [w430 w457 w474 w493 w515 w532] -> w425
        selector: w422 -> [w431 _ _ _ _ _]
        tunnel: [w429 main_prog_state."AI" main_prog_state."DI" main_prog_state."SendAItoScada" main_prog_state."Exit" main_prog_state."Read_AI_Param"] -> w423
        tunnel: [_ _ _ _ _ TRUE] -> w421
        tunnel: [w428 w451 w471 w490 w508 w531] -> w420
        frame Default {
          n124 = Increment(x=w431) -> (x+1=w429:T5)
        }
        frame "Timers" {
          # "to u=UNIX epoch"
          # "to u=UNIX epoch"
          # "to u=UNIX epoch"
          # "Mac HFS+ (ms)"
          n125 = flat-sequence {
            tunnel: [w469] -> w463
            tunnel: [w468] -> w458
            tunnel: w462 -> [w467]
            frame #0 {
              n126 = Get Date/Time In Seconds() -> (seconds since 1Jan1904=w469:timestamp)
              n127 = Bundle By Name(cluster=w467, "current time"=w469) -> (w468:T8)
            }
          }
          n128 = To Double Precision Float(number=w463) -> (double precision float=w434:dbl)
          n129 = Multiply(x=w434, y=0.1) -> (x*y=w439:dbl)
          n130 = Multiply(x=w434, y=1.157407407407407e-05) -> (x*y=w436:dbl)
          n131 = Round Toward -Infinity(1:w434) -> (0:w433:dbl)
          n132 = Round Toward -Infinity(1:w439) -> (0:w438:dbl)
          n133 = Round Toward -Infinity(1:w436) -> (0:w437:dbl)
          n134 = To Unsigned Quad Integer(1:w438) -> (0:w443:u64)
          n135 = To Unsigned Quad Integer(1:w433) -> (0:w432:u64)
          n136 = To Unsigned Quad Integer(1:w437) -> (0:w441:u64)
          n137 = Subtract(x=w432, y=u64 2082844800) -> (x-y=w435:u64)
          n138 = Subtract(x=w443, y=u64 208284480) -> (x-y=w442:u64)
          n139 = Subtract(x=w441, y=u64 24107) -> (x-y=w440:u64)
          n140 = Multiply(x=w435, y=u64 1000) -> (x*y=w460:u64)
          n141 = Multiply(x=w442, y=u64 10000) -> (x*y=w449:u64)
          n142 = Multiply(x=w440, y=u64 86400000) -> (x*y=w452:u64)
          n143 = feedback #2(w460) -> (w461:u64)
          n144 = feedback-in #2(w460) -> ()
          n145 = feedback #3(w449) -> (w448:u64)
          n146 = feedback-in #3(w449) -> ()
          n147 = feedback #4(w452) -> (w453:u64)
          n148 = feedback-in #4(w452) -> ()
          n149 = Not Equal?(x=w460, y=w461) -> (x != y?=w459:bool)
          n150 = Not Equal?(x=w449, y=w448) -> (x != y?=w444:bool)
          n151 = Not Equal?(x=w452, y=w453) -> (x != y?=w450:bool)
          n152 = Bundle By Name(cluster=w458, "Timer_1s"=w459, "Timer_10s"=w444, "Timer_1day"=w450) -> (w457:T8)
        }
        frame "AI" {
          # "AI"
          n153 = Unbundle By Name(w476) -> ("MBs"=w472:refnum<class "Modbus Master CR.lvclass">[])
          n154 = call "Read connects.vi"("error in (no error)"=w475, "MBs"=w472) -> ("error out"=w473:errorcluster, "MBs out"=w470:refnum<class "Modbus Master CR.lvclass">[])  [unwired: 7 in, 1 out]
          n155 = local read "output Flags"() -> (w478:T2)
          n156 = Unbundle By Name(w478) -> ("param handling"=w477:bool)
          n157 = for {
            tunnel: w470 -> [w488] mode=indexing
            shift-right: [w482] -> w471
            shift-left: w473 -> [w481]
            tunnel: [w480] -> _ mode=indexing
            n158 = call "Read Data Model.vi"("error in (no error)"=w481, "MB_TCP in"=w488) -> ("error out"=w487:errorcluster, "Data Model"=w489:refnum<class "Device Data Model.lvclass">, "MB_TCP out"=w486:refnum<class "Modbus Master CR.lvclass">)  [unwired: 7 in]
            n159 = call "Read N channel.vi"("error in (no error)"=w487, "MB_v2 in"=w486) -> ("error out"=w483:errorcluster, "N channel"=w485:T22)  [unwired: 7 in, 1 out]
            n160 = Unbundle By Name(w485) -> ("N AI channel"=w484:u16)
            n161 = call-dynamic "Read Holding Registers.vi"("error in"=w483, "number of registers"=w484, "device data model in"=w489) -> ("error out"=w482:errorcluster, "data"=w480:u16[])  [unwired: 6 in, 1 out]
          }
          n162 = Not(x=w477) -> ()  [unwired: 1 out]
        }
        frame "DI" {
          # "DI"
          n163 = local read "output Flags"() -> (w496:T2)
          n164 = Unbundle By Name(w496) -> ("param handling"=w495:bool)
          n165 = Unbundle By Name(w494) -> ("MBs"=w492:refnum<class "Modbus Master CR.lvclass">[])
          n166 = Not(x=w495) -> ()  [unwired: 1 out]
          n167 = for {
            tunnel: w492 -> [w506] mode=indexing
            shift-right: [w500] -> w490
            shift-left: w491 -> [w499]
            tunnel: [w498] -> _ mode=indexing
            n168 = call "Read Data Model.vi"("error in (no error)"=w499, "MB_TCP in"=w506) -> ("error out"=w505:errorcluster, "Data Model"=w507:refnum<class "Device Data Model.lvclass">, "MB_TCP out"=w504:refnum<class "Modbus Master CR.lvclass">)  [unwired: 7 in]
            n169 = call "Read N channel.vi"("error in (no error)"=w505, "MB_v2 in"=w504) -> ("error out"=w501:errorcluster, "N channel"=w503:T22)  [unwired: 7 in, 1 out]
            n170 = Unbundle By Name(w503) -> ("N DI channel"=w502:u16)
            n171 = call-dynamic "Read Discrete Inputs.vi"("error in"=w501, "number of inputs"=w502, "device data model in"=w507) -> ("error out"=w500:errorcluster, "data"=w498:bool[])  [unwired: 6 in, 1 out]
          }
        }
        frame "Outputs" {
          # "Outputs"
          n172 = Unbundle By Name(w514) -> ("MBs"=w513:refnum<class "Modbus Master CR.lvclass">[])
          n173 = Unbundle By Name(w515) -> ()  [unwired: 1 out]
          n174 = for {
            tunnel: w513 -> [w523] mode=indexing
            shift-right: [w521] -> w509
            shift-left: w512 -> [w522]
            tunnel: "AOint" -> [w519] mode=indexing
            n175 = call "Read Data Model.vi"("error in (no error)"=w522, "MB_TCP in"=w523) -> ("error out"=w520:errorcluster, "Data Model"=w518:refnum<class "Device Data Model.lvclass">)  [unwired: 7 in, 1 out]
            n176 = call-dynamic "Write Multiple Registers.vi"("error in"=w520, "register values"=w519, "starting address"=u16 0, "device data model in"=w518) -> ("error out"=w521:errorcluster)  [unwired: 6 in, 1 out]
          }
          n177 = for {
            tunnel: w513 -> [w530] mode=indexing
            shift-right: [w526] -> w508
            shift-left: w509 -> [w525]
            tunnel: "DO2D" -> [w524] mode=indexing
            n178 = call "Read Data Model.vi"("error in (no error)"=w525, "MB_TCP in"=w530) -> ("error out"=w529:errorcluster, "Data Model"=w528:refnum<class "Device Data Model.lvclass">)  [unwired: 7 in, 1 out]
            n179 = call-dynamic "Write Multiple Coils.vi"("error in"=w529, "coils"=w524, "starting address"=u16 0, "device data model in"=w528) -> ("error out"=w526:errorcluster)  [unwired: 6 in, 1 out]
          }
        }
        frame "Exit" {
        }
      }
    }
    n180 = local read "output Flags"() -> (w411:T2)
    n181 = Unbundle By Name(w411) -> ("main prog stopped"=w410:bool)
    n182 = node-c288(w416, "tick") -> ()  [unwired: 1 out]
  }
  n183 = node-c288(w18) -> (w17:errorcluster)
  n184 = flat-sequence {
    tunnel: w17 -> [w544]
    tunnel: [w544] -> w6
    frame #0 {
      n185 = local read "input Flags"() -> (w542:T1)
      n186 = Bundle By Name(cluster=w542, "main prog started"=FALSE) -> (w543:T1)
      n187 = local write "input Flags"(w543) -> ()
    }
  }
  n188 = Merge Errors(w7, w6) -> (w5:errorcluster)  [unwired: 3 in]
  n189 = flat-sequence {
    tunnel: w2 -> [w548]
    tunnel: _ -> [w546]
    tunnel: w5 -> [w547]
    tunnel: [w546] -> w4
    tunnel: [w545] -> w3
    tunnel: [w665] -> w15
    tunnel: w4 -> [w667]
    tunnel: w3 -> [w666]
    frame #0 {
      n190 = while "Close" {
        shift-right: [w554] -> _
        shift-left: close_state."QN_state notifier" ("Init_state") -> [w555]
        tunnel: w548 -> [w552]
        shift-right: [w550] -> w545
        shift-left: w547 -> [w551]
        stop <- w553 stop-if-true
        n191 = case shown="Default" w555 {
          selector: w555 -> [_ _ _ _ _ _ _ _ _ _ _ _ _ _ _ _ _ _ w664]
          tunnel: [close_state."QN_control_queue" close_state."ALR notifires" close_state."ALR" close_state."DO notifires" close_state."DO" close_state."AO notifires" close_state."AO" close_state."DI notifres" close_state."DI" close_state."AI notifires" close_state."AI" close_state."OPC" close_state."Param" close_state."SaveMessageProg" close_state."KFM DadaRef" close_state."KFM Registers" close_state."Exit" close_state."OPC" w663] -> w554
          tunnel: [_ _ _ _ _ _ _ _ _ _ _ _ _ _ _ _ _ TRUE _] -> w553
          tunnel: w552 -> [w556 w562 w573 w579 w585 w591 w597 w603 w609 w615 w621 w627 w633 w639 w645 w653 _ _ _]
          tunnel: w551 -> [w558 w564 w571 w577 w583 w589 w595 w601 w607 w613 w619 w625 w630 w637 w643 w651 w656 w660 w662]
          tunnel: [w557 w563 w570 w576 w582 w588 w594 w600 w606 w612 w618 w624 w628 w636 w642 w650 w656 w660 w662] -> w550
          frame "QN_state notifier" {
            n192 = Unbundle By Name(w556) -> ("QN_state notifier"=w560)
            n193 = Release Notifier(notifier=w560) -> (error out=w559:errorcluster)  [unwired: 2 in, 2 out]
            n194 = Merge Errors(w559, w558) -> (w557:errorcluster)
          }
          frame "QN_control_queue" {
            n195 = Unbundle By Name(w562) -> ("QN_control queue"=w566)
            n196 = Release Queue(queue=w566) -> (error out=w565:errorcluster)  [unwired: 2 in, 2 out]
            n197 = Merge Errors(w565, w564) -> (w563:errorcluster)
          }
          frame "ALR notifires" {
            n198 = Unbundle By Name(w573) -> ("ALR notifier"=w569)
            n199 = Release Notifier(notifier=w569) -> (error out=w568:errorcluster)  [unwired: 2 in, 2 out]
            n200 = Merge Errors(w568, w571) -> (w570:errorcluster)
          }
          frame "ALR" {
            n201 = Unbundle By Name(w579) -> ("Alarms"=w575)
            n202 = call "ALR destroy.vi"("Alarms in"=w575) -> ("error out"=w574:errorcluster)  [unwired: 10 in]
            n203 = Merge Errors(w574, w577) -> (w576:errorcluster)
          }
          frame "DO notifires" {
            n204 = Unbundle By Name(w585) -> ("DO notifier"=w581)
            n205 = Release Notifier(notifier=w581) -> (error out=w580:errorcluster)  [unwired: 2 in, 2 out]
            n206 = Merge Errors(w580, w583) -> (w582:errorcluster)
          }
          frame "DO" {
            n207 = Unbundle By Name(w591) -> ("Enums.DO"=w587:string[])
            n208 = call "Close DO.vi"("DO in"=w587) -> ("error out"=w586:errorcluster)  [unwired: 10 in]
            n209 = Merge Errors(w586, w589) -> (w588:errorcluster)
          }
          frame "AO notifires" {
            n210 = Unbundle By Name(w597) -> ("AO notifier"=w593)
            n211 = Release Notifier(notifier=w593) -> (error out=w592:errorcluster)  [unwired: 2 in, 2 out]
            n212 = Merge Errors(w592, w595) -> (w594:errorcluster)
          }
          frame "AO" {
            n213 = Unbundle By Name(w603) -> ("Enums.AO"=w599:string[])
            n214 = call "Close AO.vi"("AO in"=w599) -> ("error out"=w598:errorcluster)  [unwired: 10 in]
            n215 = Merge Errors(w598, w601) -> (w600:errorcluster)
          }
          frame "DI notifres" {
            n216 = Unbundle By Name(w609) -> ("DI notifier"=w605)
            n217 = Release Notifier(notifier=w605) -> (error out=w604:errorcluster)  [unwired: 2 in, 2 out]
            n218 = Merge Errors(w604, w607) -> (w606:errorcluster)
          }
          frame "DI" {
            n219 = Unbundle By Name(w615) -> ("Enums.DI"=w611:string[])
            n220 = call "Close DI.vi"("DI in"=w611) -> ("error out"=w610:errorcluster)  [unwired: 10 in]
            n221 = Merge Errors(w610, w613) -> (w612:errorcluster)
          }
          frame "AI notifires" {
            n222 = Unbundle By Name(w621) -> ("AI notifier"=w617)
            n223 = Release Notifier(notifier=w617) -> (error out=w616:errorcluster)  [unwired: 2 in, 2 out]
            n224 = Merge Errors(w616, w619) -> (w618:errorcluster)
          }
          frame "AI" {
            n225 = Unbundle By Name(w627) -> ("Enums.AI"=w623:string[])
            n226 = call "AI close.vi"("AI in"=w623) -> ("error out"=w622:errorcluster)  [unwired: 10 in]
            n227 = Merge Errors(w622, w625) -> (w624:errorcluster)
          }
          frame "OPC" {
            n228 = Unbundle By Name(w633) -> ("OPC UA"=w632)
            n229 = call "Close Server.vi"("OPC UA"=w632) -> ("error out"=w629:errorcluster)  [unwired: 10 in]
            n230 = Merge Errors(w629, w630) -> (w628:errorcluster)
          }
          frame "Param" {
            n231 = Unbundle By Name(w639) -> ("Param"=w635)
            n232 = call "Close Param.vi"("Param in"=w635) -> ("error out"=w634:errorcluster)  [unwired: 10 in]
            n233 = Merge Errors(w634, w637) -> (w636:errorcluster)
          }
          frame "SaveMessageProg" {
            n234 = Unbundle By Name(w645) -> ("SMPs"=w641)
            n235 = for {
              tunnel: w641 -> [w647]
              tunnel: [w646] -> w640 mode=indexing
              n236 = call "Close.vi"("MB in"=w647) -> ("error out"=w646:errorcluster)  [unwired: 10 in]
            }
            n237 = Merge Errors(w640, w643) -> (w642:errorcluster)
          }
          frame "KFM DadaRef" {
            n238 = Unbundle By Name(w653) -> ("MBs"=w649:refnum<class "Modbus Master CR.lvclass">[])
            n239 = for {
              tunnel: w649 -> [w655] mode=indexing
              tunnel: [w654] -> w648 mode=indexing
              n240 = call-dynamic "Shutdown.vi"("MB in"=w655) -> ("error out"=w654:errorcluster)  [unwired: 10 in]
            }
            n241 = Merge Errors(w648, w651) -> (w650:errorcluster)
          }
          frame "KFM StatusRef" {
          }
          frame "Exit" {
            n242 = local write "output Flags"(T2 {"parameters readed "=FALSE, "AI readed"=FALSE, "DI readed"=FALSE, "AO readed"=FALSE, "DO readed"=FALSE, "ALR readed"=FALSE, "read I/O started"=FALSE, "param handling"=FALSE, "ALR handling"=FALSE, "write database stopped"=FALSE, "main prog stopped"=FALSE} ("output Flags")) -> ()
          }
          frame Default {
            n243 = Increment(x=w664) -> (x+1=w663:T23)
          }
        }
      }
    }
    frame #1 {
      n244 = call "Release message Queues.vi"("Messages"=w667) -> ("error out"=w668:errorcluster)  [unwired: 10 in]
      n245 = Merge Errors(w668, w666) -> (w665:errorcluster)  [unwired: 1 in]
    }
  }
  "comm error" <- w15
